vi "Exercise1.18-Random Noise Display.vi"() -> ()   [LabVIEW 2013]
panel:
  out "Waveform Graph":waveform(dbl)(graph)
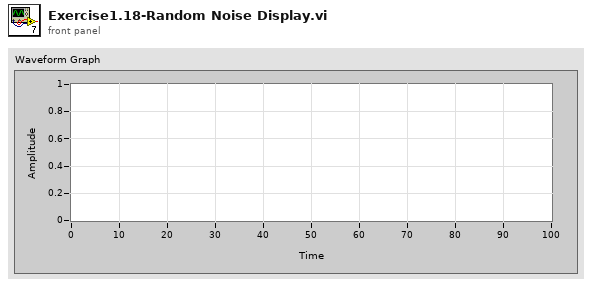
[diagram p1: front panel]
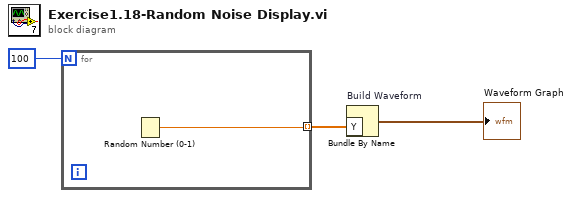
[diagram p0: block diagram]
diagram:
  n1 = for {
    N: 100 -> [_]
    tunnel: [w4] -> w2 mode=indexing
    n2 = Random Number (0-1)() -> (number: 0 to 1=w4:dbl)
  }
  n3 = Bundle By Name "Build Waveform"("Y"=w2) -> (→"Waveform Graph":waveform(dbl))  [unwired: 1 in]
